vi "Unload.vi"(8 "error in (no error)":errorcluster, 11 "Channel in":refnum<data-value>) -> (0 "error out":errorcluster, 3 "Channel out":refnum<data-value>)   [LabVIEW 2020, in "G-Audio.lvlib" / "Channel.lvclass"]
uses:
  Channel.lvclass
  Mixer/Controls/Mixer Audio Data Type.ctl
  Mixer/Mixer.lvclass
  93f27375-c45a-4c4b-923f-bd89424912f9.vi
  60d18774-9d30-42b4-b70e-efb8e1f052d1.vi
  Controls/Channel State.ctl
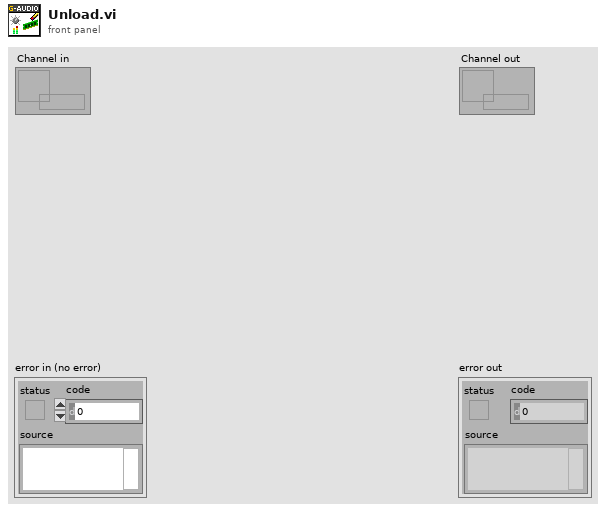
[diagram p1: front panel]
types:
  T1 = typedef "G-Audio.lvlib/Channel.lvclass/Channel State.ctl" = enum16{"Empty", "Error", "Loading", "Loaded", "Stopped", "Paused", "Playing", "Retrigger"}
  T2 = typedef "G-Audio.lvlib/Mixer.lvclass/Mixer Audio Data Type.ctl" = i16[][]
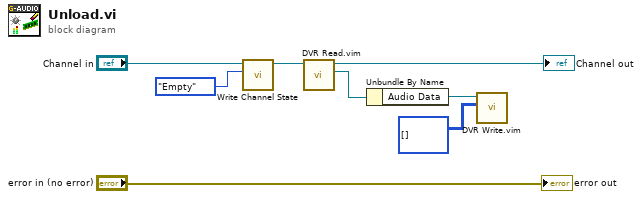
[diagram p0: block diagram]
diagram:
  n1 = call "Write Channel State.vi"("State"=Channel_State."Empty", "Channel in"="Channel in") -> ("Channel out"=w3:refnum<data-value>)  [unwired: 8 in, 1 out]
  n2 = call "DVR Read.vim"("DVR In"=w3) -> ("Data"=w6:refnum<class "Channel.lvclass">, "DVR Out"=→"Channel out":refnum<data-value>)  [unwired: 9 in]
  n3 = Unbundle By Name(w6) -> ("Audio Data"=w8:refnum<data-value>)
  n4 = call "DVR Write.vim"("Data"=T2 [] ("Audio Data Type"), "DVR In"=w8) -> ()  [unwired: 9 in, 1 out]
  "error out" <- "error in (no error)"
